vi "FahrprofileSchreiben.vi"() -> ()   [LabVIEW 2023]
doc: "Converts an array of data to a row of tab-separated columns, prepends the timestamp column, and terminates each row with the end of line character."
panel:
  in  "stop":bool
  in  "Datei (Name.txt)":path
  in  "Geschwindigkeit":dbl
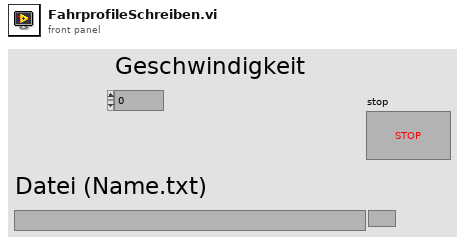
[diagram p1: front panel]
types:
  T1 = enum16{"open", "replace", "create", "open or create", "replace or create", "replace or create with confirmation"}
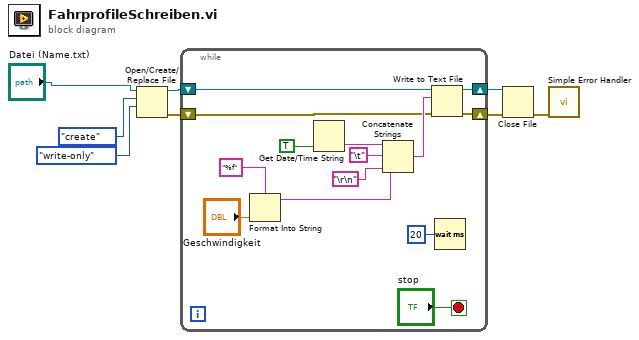
[diagram p0: block diagram]
diagram:
  n1 = Open/Create/Replace File(file path (use dialog)="Datei (Name.txt)", operation (0:open)=T1."create", access (0:read/write)=enum16{"read/write", "read-only", "write-only"}."write-only") -> (refnum out=w4:refnum<file>, error out=w5:errorcluster)  [unwired: 1 in, 3 out]
  n2 = while {
    shift-right: [w12] -> w3
    shift-left: w5 -> [w17]
    shift-right: [w11] -> w2
    shift-left: w4 -> [w16]
    stop <- "stop" stop-if-true
    n3 = Format Into String(format string="%f", "Geschwindigkeit") -> (resulting string=w22:string)  [unwired: 2 in, 1 out]
    n4 = Get Date/Time String(want seconds? (F)=TRUE) -> (time string=w21:string)  [unwired: 2 in, 1 out]
    n5 = Concatenate Strings(w21, "\t" ("Tab"), w22, "\r\n") -> (w20:string)
    n6 = Write to Text File(file (use dialog)=w16, text=w20, error in=w17) -> (refnum out=w11:refnum<file>, error out=w12:errorcluster)  [unwired: 1 in, 1 out]
    n7 = Wait (ms)(milliseconds to wait=u32 20) -> ()  [unwired: 1 out]
  }
  n8 = Close File(refnum=w2, error in=w3) -> (error out=w8:errorcluster)  [unwired: 1 out]
  n9 = call <vilib>:"Simple Error Handler.vi"("error in (no error)"=w8) -> ()  [unwired: 1 in, 8 out]
